vi "Thorlabs-Shutter-Toggle.vi"(8 "Device in Y":refnum<k24>, 10 "Delay":dbl, 11 "Device in X":refnum<k24>) -> (0 "Device out Y":refnum<k24>, 3 "Device out X":refnum<k24>)   [LabVIEW 2014]
uses:
  C:/UserLab/andre/GITs/andretec/Thorlabs-Vector-Move/kinesisTec/Kinesis/Thorlabs.MotionControl.TCube.DCServoCLI.dll
  Kinesis/Thorlabs.MotionControl.TCube.DCServoCLI.dll
  motorsGlobalVar.vi
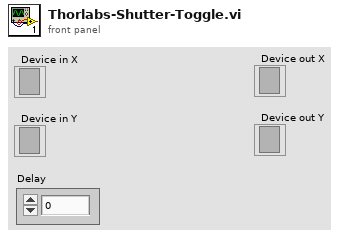
[diagram p1: front panel]
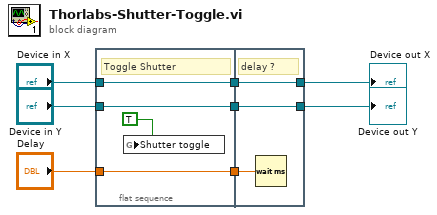
[diagram p0: block diagram]
diagram:
  n1 = flat-sequence {
    tunnel: "Device in X" -> [w11]
    tunnel: "Device in Y" -> [w10]
    tunnel: [w11] -> w8
    tunnel: [w10] -> w7
    tunnel: "Delay" -> [w9]
    tunnel: [w9] -> w1
    tunnel: w8 -> [w15]
    tunnel: [w15] -> w5
    tunnel: w7 -> [w14]
    tunnel: [w14] -> w6
    tunnel: w1 -> [w13]
    frame #0 {
      # "Toggle Shutter"
      n2 = global write "motorsGlobalVar.vi" "Shutter toggle"(TRUE ("Shutter toggle")) -> ()
    }
    frame #1 {
      # "delay ?"
      n3 = Wait (ms)(milliseconds to wait=w13) -> ()  [unwired: 1 out]
    }
  }
  "Device out Y" <- w6
  "Device out X" <- w5
